vi "calculator_Project.vi"() -> ()   [LabVIEW 2020]
panel:
  out "Result":string
  in  "Cluster":T1
  # "CASIO"
  # "CT-501"
  # "Basic Calculator"
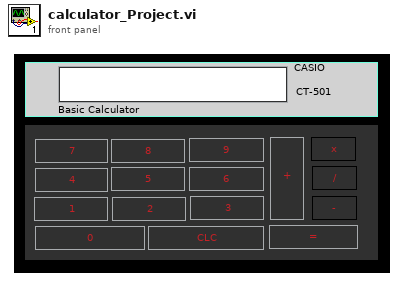
[diagram p1: front panel]
types:
  T1 = cluster{"1":bool, "2":bool, "3":bool, "Add":bool, "4":bool, "5":bool, "6":bool, "Sub":bool, "7":bool, "8":bool, "9":bool, "Mul":bool, "Clear":bool, "0":bool, "Equal":bool, "Div":bool}
  T2 = enum16{"No Function", "Add", "Sub", "Mul", "Div"}
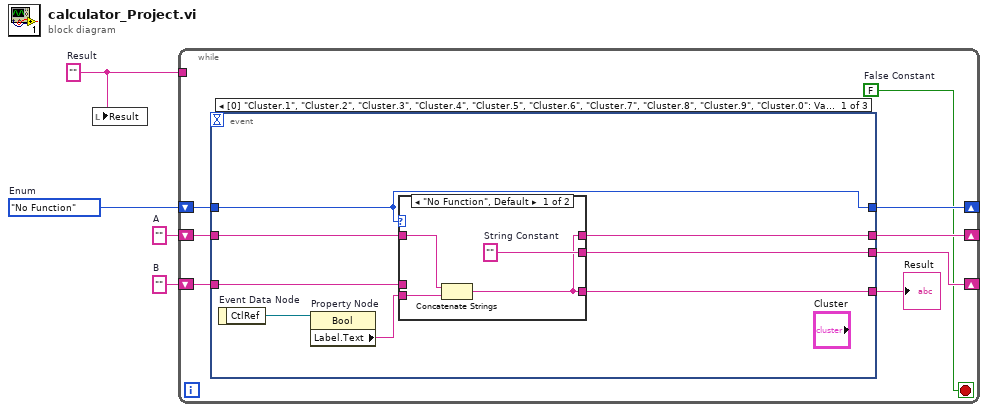
[diagram p0: block diagram]
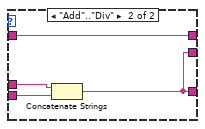
[diagram p2: hidden frame]
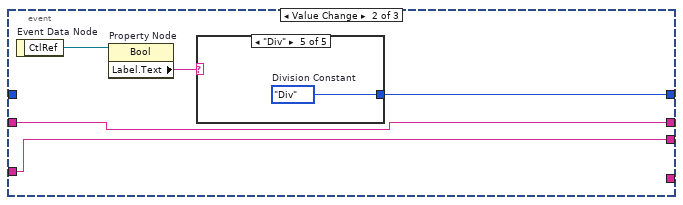
[diagram p3: hidden frame]
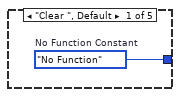
[diagram p4: hidden frame]
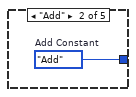
[diagram p5: hidden frame]
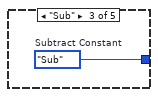
[diagram p6: hidden frame]
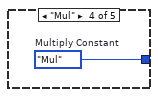
[diagram p7: hidden frame]
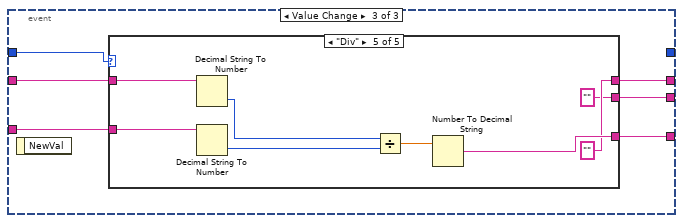
[diagram p8: hidden frame]
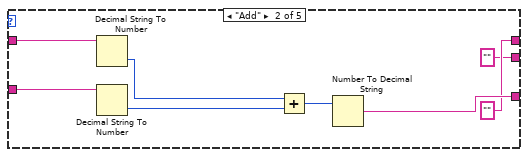
[diagram p10: hidden frame]
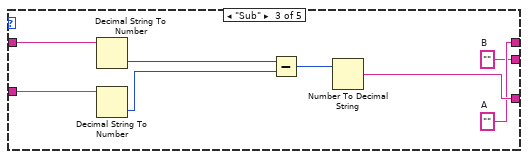
[diagram p11: hidden frame]
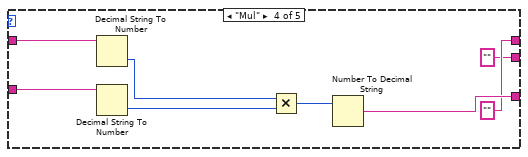
[diagram p12: hidden frame]
diagram:
  w1 = ""  # Result
  w2 = ""  # B
  w3 = ""  # A
  w4 = T2."No Function"  # Enum
  n1 = local write "Result"(w1) -> ()
  n2 = while {
    shift-right: [w8] -> _
    shift-left: w3 -> [w12]
    shift-right: [w7] -> _
    shift-left: w2 -> [w11]
    shift-right: [w9] -> _
    shift-left: w4 -> [w10]
    tunnel: w1 -> [_]
    stop <- w5 stop-if-true
    w5 = FALSE  # False Constant
    n3 = event shown="[0] \"Cluster.1\", \"Cluster.2\", \"Cluster.3\", \"Cluster.4\", \"Cluster.5\", \"Cluster.6\", \"Cluster.7\", \"Cluster.8\", \"Cluster.9\", \"Cluster.0\": Value Change" {
      selector: _ -> [_ _ _]
      dyn-events: _ -> [_ _ _]
      timeout: _ -> [_ _ _]
      tunnel: w12 -> [w18 w33 w43]
      tunnel: w11 -> [w14 w32 w41]
      tunnel: w10 -> [w19 _ w44]
      tunnel: [w19 w29 _] -> w9
      tunnel: [w16 w33 w42] -> w8
      tunnel: [w15 w32 w40] -> w7
      tunnel: [w13 _ w39] -> w6
      event "Cluster.1", "Cluster.2", "Cluster.3", "Cluster.4", "Cluster.5", "Cluster.6", "Cluster.7", "Cluster.8", "Cluster.9", "Cluster.0": Value Change {
        n4 = event-data "Event Data Node"() -> ("CtlRef"=w20:refnum<vi>)  [unwired: 1 in]
        n5 = property on="Property Node" class="Bool"(reference=w20) -> ("Label.Text"=w17:string)  [unwired: 1 in, 2 out]
        n6 = case shown="\"No Function\", Default" w19 {
          tunnel: w18 -> [w24 w25]
          tunnel: w17 -> [w23 w28]
          tunnel: [w21 w25] -> w16
          tunnel: [w22 w26] -> w15
          tunnel: w14 -> [_ w27]
          tunnel: [w21 w26] -> w13
          frame "No Function", Default {
            w22 = ""  # String Constant
            n7 = Concatenate Strings "Concatenate Strings"(w24, w23) -> (w21:string)
          }
          frame "Add".."Div" {
            n8 = Concatenate Strings "Concatenate Strings"(w27, w28) -> (w26:string)
          }
        }
      }
      event "Cluster.Clear", "Cluster.Sub", "Cluster.Mul", "Cluster.Div", "Cluster.Add": Value Change {
        n9 = event-data "Event Data Node"() -> ("CtlRef"=w31:refnum<vi>)  [unwired: 1 in]
        n10 = property on="Property Node" class="Bool"(reference=w31) -> ("Label.Text"=w30:string)  [unwired: 1 in, 2 out]
        n11 = case shown="\"Div\"" w30 {
          tunnel: [w34 w35 w36 w37 w38] -> w29
          frame "Clear ", Default {
            w34 = T2."No Function"  # No Function Constant
          }
          frame "Add" {
            w35 = T2."Add"  # Add Constant
          }
          frame "Sub" {
            w36 = T2."Sub"  # Subtract Constant
          }
          frame "Mul" {
            w37 = T2."Mul"  # Multiply Constant
          }
          frame "Div" {
            w38 = T2."Div"  # Division Constant
          }
        }
      }
      event "Cluster.Equal": Value Change {
        n12 = event-data() -> ()  [unwired: 1 in, 1 out]
        n13 = case shown="\"Div\"" w44 {
          tunnel: [w45 "" ("A") w56 "" ("A") "" ("A")] -> w42
          tunnel: w43 -> [w45 w54 w62 w70 w78]
          tunnel: w41 -> [w46 w53 w61 w69 w77]
          tunnel: [w46 "" ("B") w55 "" ("B") "" ("B")] -> w40
          tunnel: [w45 w49 w57 w65 w73] -> w39
          frame "No Function", Default {
          }
          frame "Add" {
            n14 = Decimal String To Number(string=w54) -> (number=w52:i32)  [unwired: 2 in, 1 out]
            n15 = Decimal String To Number(string=w53) -> (number=w51:i32)  [unwired: 2 in, 1 out]
            n16 = Add(x=w52, y=w51) -> (x+y=w50:i32)
            n17 = Number To Decimal String(number=w50) -> (decimal integer string=w49:string)  [unwired: 1 in]
          }
          frame "Sub" {
            w55 = ""  # B
            w56 = ""  # A
            n18 = Decimal String To Number(string=w62) -> (number=w60:i32)  [unwired: 2 in, 1 out]
            n19 = Decimal String To Number(string=w61) -> (number=w59:i32)  [unwired: 2 in, 1 out]
            n20 = Subtract(x=w60, y=w59) -> (x-y=w58:i32)
            n21 = Number To Decimal String(number=w58) -> (decimal integer string=w57:string)  [unwired: 1 in]
          }
          frame "Mul" {
            n22 = Decimal String To Number(string=w70) -> (number=w68:i32)  [unwired: 2 in, 1 out]
            n23 = Decimal String To Number(string=w69) -> (number=w67:i32)  [unwired: 2 in, 1 out]
            n24 = Multiply(x=w68, y=w67) -> (x*y=w66:i32)
            n25 = Number To Decimal String(number=w66) -> (decimal integer string=w65:string)  [unwired: 1 in]
          }
          frame "Div" {
            n26 = Decimal String To Number(string=w78) -> (number=w76:i32)  [unwired: 2 in, 1 out]
            n27 = Decimal String To Number(string=w77) -> (number=w75:i32)  [unwired: 2 in, 1 out]
            n28 = Divide(x=w76, y=w75) -> (x/y=w74:dbl)
            n29 = Number To Decimal String(number=w74) -> (decimal integer string=w73:string)  [unwired: 1 in]
          }
        }
      }
    }
    "Result" <- w6
  }
